vi "Interface.vi"(9 "EventsIn":T1, 10 "Events":T2) -> ()   [LabVIEW 2014, in "GCMSettingsScreen.lvlib" / "GCMSettingsScreen.lvclass"]
uses:
  GCMSettingsScreen.lvclass
  _LVCMPlugin/GCMPlugin_EventsOut.ctl
  _LVCMPlugin/GCMPlugin_EventsIn.ctl
  Command.ctl
  GCMConfigurationManager/GCMConfigurationManager.lvclass
  GCMPlugin/GCMPlugin.lvclass
panel:
  in  "Open GCM window when LV project opens":bool
  out "SettingsLabel":string="GCM Settings"
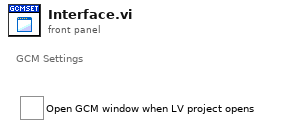
[diagram p1: front panel]
types:
  T1 = typedef "GCMPlugin.lvclass/GCMPlugin_EventsIn.ctl" = cluster{"Stop":refnum<user-event>, "ItemSelected":refnum<user-event>, "ItemDeselected":refnum<user-event>, "PluginActivated":refnum<user-event>, "PluginDeactivated":refnum<user-event>}
  T2 = typedef "GCMPlugin.lvclass/GCMPlugin_EventsOut.ctl" = cluster{"ItemEdited":refnum<user-event>}
  T3 = typedef "GCMSettingsScreen.lvlib/GCMSettingsScreen.lvclass/Command.ctl" = enum16{"Stop"}
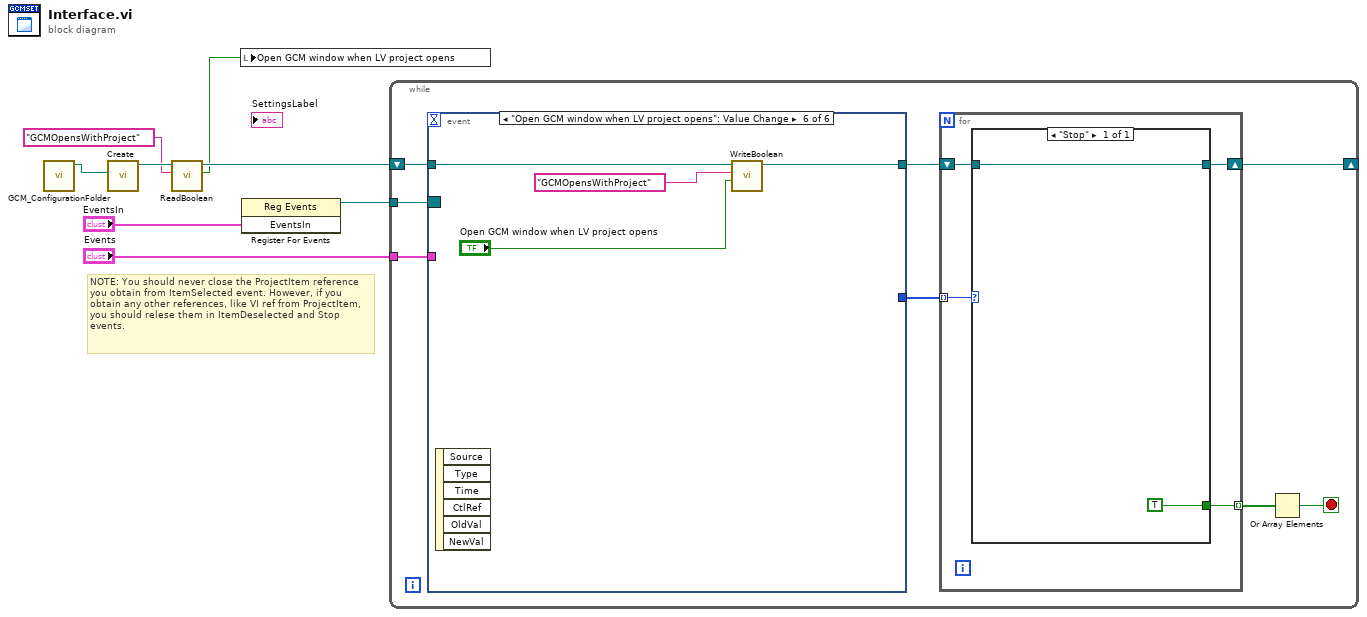
[diagram p0: block diagram]
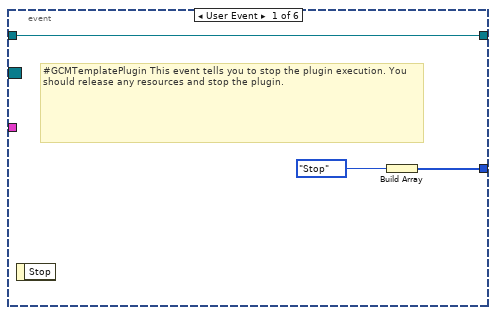
[diagram p2: hidden frame]
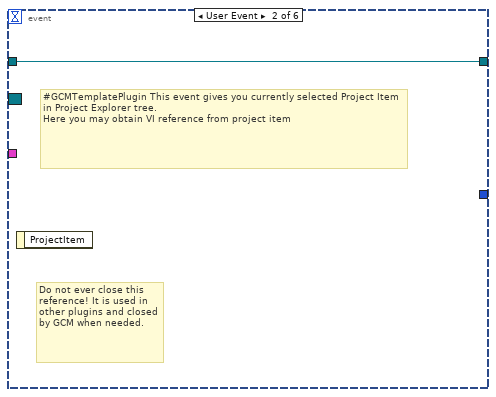
[diagram p3: hidden frame]
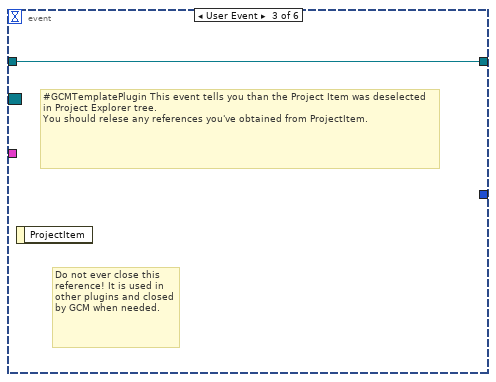
[diagram p4: hidden frame]
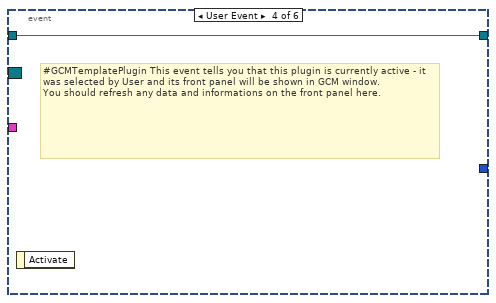
[diagram p5: hidden frame]
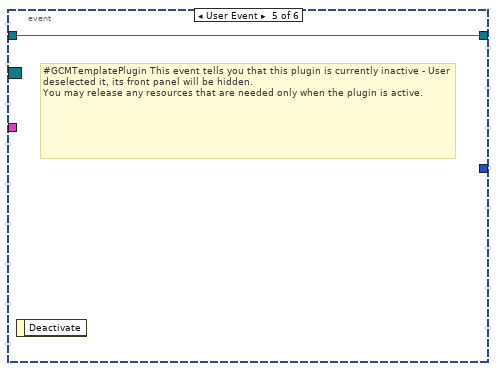
[diagram p6: hidden frame]
diagram:
  # "NOTE: You should never close the ProjectItem reference you obtain from ItemSelected event. However, if you obtain any other references, like VI ref from ProjectItem, you should relese them in ItemDeselected and Stop events."
  n1 = call "GCM_ConfigurationFolder.vi"() -> ("ConfigurationFolder"=w1:path)  [unwired: 11 in]
  n2 = call "Create.vi"("ConfigurationFolder"=w1) -> ("GCMConfigurationManager out"=w5:refnum<class "GCMConfigurationManager.lvclass">)  [unwired: 9 in, 1 out]
  n3 = call "ReadBoolean.vi"("Key"="GCMOpensWithProject", "GCMConfigurationManager in"=w5) -> ("Value"=w3:bool, "GCMConfigurationManager out"=w4:refnum<class "GCMConfigurationManager.lvclass">)  [unwired: 7 in, 1 out]
  n4 = local write "Open GCM window when LV project opens"(w3) -> ()
  n5 = register-events("EventsIn") -> (reference out=w7:refnum<event-registration>)  [unwired: 2 in, 1 out]
  n6 = while {
    tunnel: w7 -> [w16]
    tunnel: "Events" -> [w15]
    shift-right: [w9] -> _
    shift-left: w4 -> [w11]
    stop <- w12 stop-if-true
    n7 = event shown="[5] \"Open GCM window when LV project opens\": Value Change" {
      selector: w16 -> [_ _ _ _ _ _]
      dyn-events: _ -> [_ _ _ _ _ _]
      timeout: _ -> [_ _ _ _ _ _]
      tunnel: w15 -> [_ _ _ _ _ _]
      tunnel: [w24 _ _ _ _ _] -> w14
      tunnel: w11 -> [w23 w26 w27 w28 w29 w33]
      tunnel: [w23 w26 w27 w28 w29 w32] -> w10
      event User Event {
        # "#GCMTemplatePlugin This event tells you to stop the plugin execution. You should release any resources and stop the plugin."
        n8 = event-data() -> ()  [unwired: 1 in, 1 out]
        n9 = Build Array(Command."Stop" ("Command")) -> (w24:T3[])
      }
      event User Event {
        # "Do not ever close this reference! It is used in other plugins and closed by GCM when needed."
        # "#GCMTemplatePlugin This event gives you currently selected Project Item in Project Explorer tree.\nHere you may obtain VI reference from project item"
        n10 = event-data() -> ()  [unwired: 1 in, 1 out]
      }
      event User Event {
        # "Do not ever close this reference! It is used in other plugins and closed by GCM when needed."
        # "#GCMTemplatePlugin This event tells you than the Project Item was deselected in Project Explorer tree.\nYou should relese any references you've obtained from ProjectItem."
        n11 = event-data() -> ()  [unwired: 1 in, 1 out]
      }
      event User Event {
        # "#GCMTemplatePlugin This event tells you that this plugin is currently active - it was selected by User and its front panel will be shown in GCM window.\nYou should refresh any data and informations on the front panel here."
        n12 = event-data() -> ()  [unwired: 1 in, 1 out]
      }
      event User Event {
        # "#GCMTemplatePlugin This event tells you that this plugin is currently inactive - User deselected it, its front panel will be hidden.\nYou may release any resources that are needed only when the plugin is active."
        n13 = event-data() -> ()  [unwired: 1 in, 1 out]
      }
      event "Open GCM window when LV project opens": Value Change {
        n14 = event-data() -> ()  [unwired: 1 in, 6 out]
        n15 = call "WriteBoolean.vi"("Value"="Open GCM window when LV project opens", "Key"="GCMOpensWithProject", "GCMConfigurationManager in"=w33) -> ("GCMConfigurationManager out"=w32:refnum<class "GCMConfigurationManager.lvclass">)  [unwired: 7 in, 1 out]
      }
    }
    n16 = for {
      tunnel: w14 -> [w20] mode=indexing
      tunnel: [w19] -> w13 mode=indexing
      shift-right: [w18] -> w9
      shift-left: w10 -> [w17]
      n17 = case shown="\"Stop\"" w20 {
        tunnel: [TRUE] -> w19
        tunnel: [w21] -> w18
        tunnel: w17 -> [w21]
        frame "Stop" {
        }
      }
    }
    n18 = Or Array Elements(Boolean array=w13) -> (logical OR=w12:bool)
  }
